vi "Load Messages and Populate Controls.vi"(8 "error in (no error)":errorcluster, 10 "Hierarchy":refnum<vi>, 11 "ListBox in":refnum<vi>) -> (0 "error out":errorcluster, 3 "Message map":map{string, T1}(c390))   [LabVIEW 2020, in "Sequencer.lvlib"]
uses:
  Sequencer.lvlib
  Controls/Ctl_MessageListElement.ctl
  PPL/HDH.ClassLoader.lvlibp
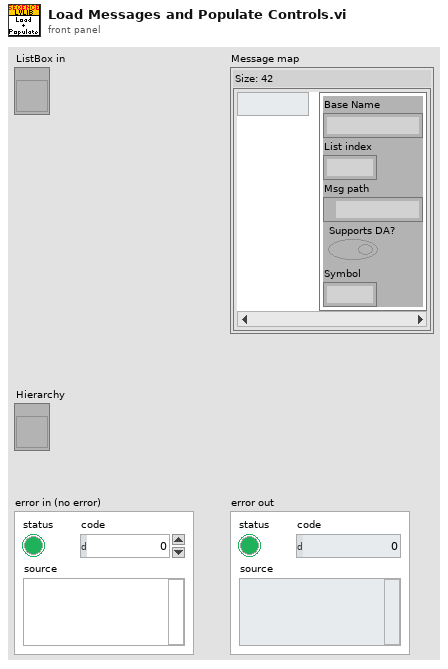
[diagram p1: front panel]
types:
  T1 = typedef "Sequencer.lvlib/Ctl_MessageListElement.ctl" = cluster{"Base Name":string, "List index":i32, "Msg path":path, "Supports DA?":bool, "Symbol":i32}
  T2 = typedef "HDH.ClassLoader.lvlibp/Ctl_Member Map.ctl" = map{string, T3}
  T3 = typedef "HDH.ClassLoader.lvlibp/HDH.ClassLoader_Member VI Info.ctl" = cluster{"qualified name":string, "path":path, "access scope":enum32{"invalid scope", "public", "private", "protected", "community"}, "is dynamic dispatch":bool}
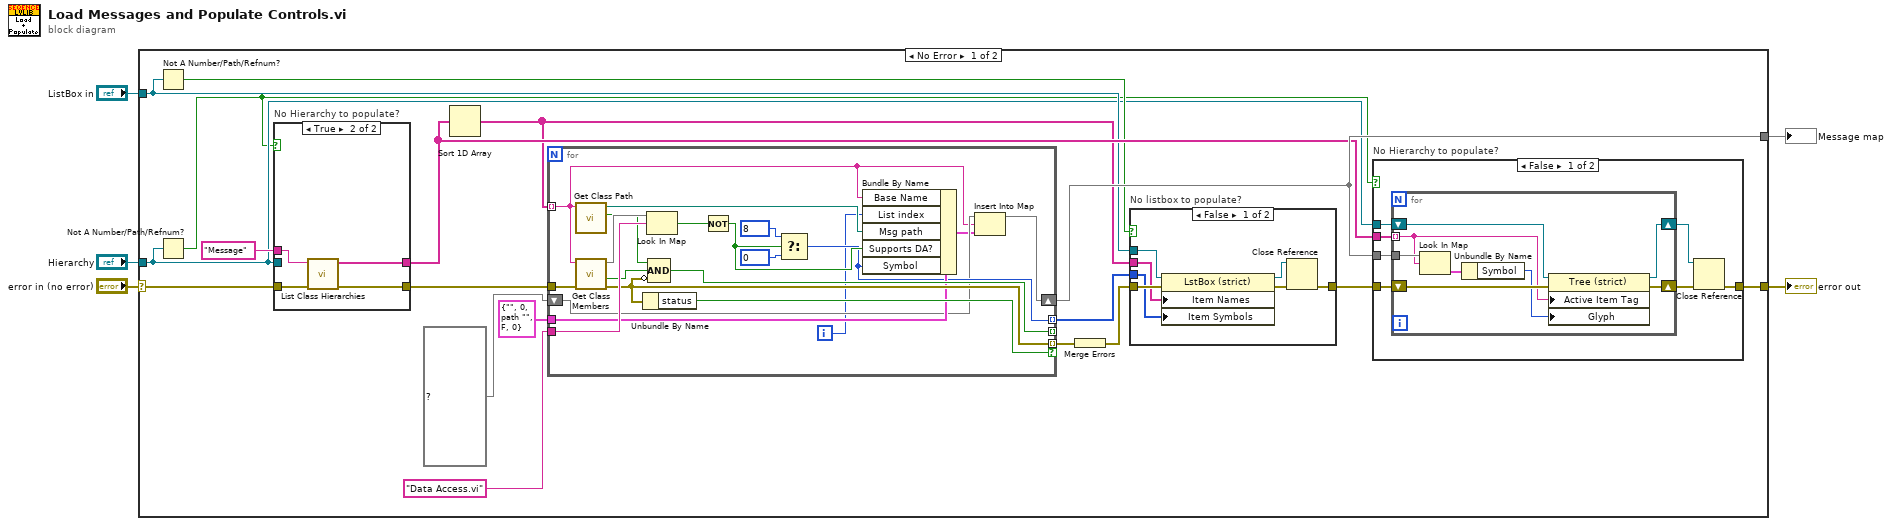
[diagram p0: block diagram]
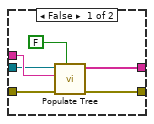
[diagram p3: hidden frame]
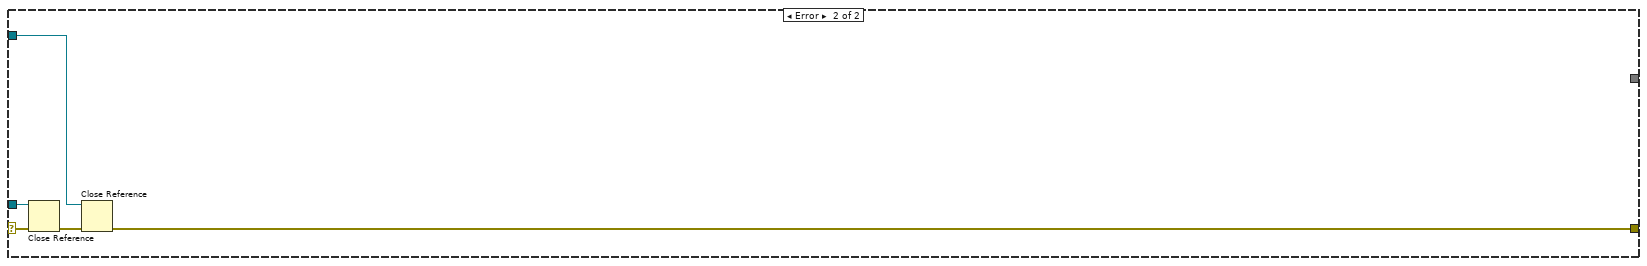
[diagram p5: hidden frame]
diagram:
  n1 = case shown="No Error" "error in (no error)" {
    selector: "error in (no error)" -> [w11 w82]
    tunnel: "Hierarchy" -> [w7 w79]
    tunnel: [w22 w81] -> w4
    tunnel: [w21 _] -> w3
    tunnel: "ListBox in" -> [w9 w78]
    frame No Error {
      n2 = Not A Number/Path/Refnum?(number/path/refnum=w9) -> (NaN/Path/Refnum?=w8:bool)
      n3 = Not A Number/Path/Refnum?(number/path/refnum=w7) -> (NaN/Path/Refnum?=w6:bool)
      n4 = case "No Hierarchy to populate?" shown="True" w6 {
        tunnel: [w44 w47] -> w20
        tunnel: [w43 w46] -> w13
        tunnel: w11 -> [w42 w49]
        tunnel: "Message" ("Hierarchy Filter(empty=all)") -> [w41 w48]
        tunnel: w7 -> [w40 _]
        frame False {
          n5 = call "Populate Tree.vi"("Close Reference?(T)"=FALSE, "error in (no error)"=w42, "Hierarchy Filter(empty=all)"=w41, "TreeControl in"=w40) -> ("error out"=w43:errorcluster, "Classes found"=w44:string[])  [unwired: 5 in, 1 out]
        }
        frame True {
          n6 = call "List Class Hierarchies.vi"("error in (no error)"=w49, "Hierarchy Filter(empty=all)"=w48) -> ("error out"=w46:errorcluster, "Classes found"=w47:string[])  [unwired: 6 in, 2 out]
        }
      }
      n7 = Sort 1D Array(array=w20) -> (sorted array=w15:string[])
      n8 = for {
        tunnel: w15 -> [w59] mode=indexing
        tunnel: w13 -> [w77]
        tunnel: "Data Access.vi" ("name or relative path") -> [w75]
        tunnel: [w70] -> w14 mode=indexing if=w73
        tunnel: [w69] -> _ mode=indexing
        tunnel: [w63] -> w16 mode=indexing
        tunnel: T1 {"Base Name"="", "List index"=0, "Msg path"=path "", "Supports DA?"=FALSE, "Symbol"=0} -> [w66]
        shift-right: [w61] -> w21
        shift-left: map{string, T1} {} ("map") -> [w62]
        i -> [w58]
        n9 = call "Get Class Path.vi"("Base Class Name"=w59) -> ("Success?"=w72:bool, "Path"=w65:path)  [unwired: 9 in]
        n10 = call "Get Class Members.vi"("error in (no error)"=w77, "Base Class Name"=w59) -> ("error out"=w70:errorcluster, "Success?"=w71:bool, "Member Map"=w76:T2)  [unwired: 7 in]
        n11 = Unbundle By Name(w70) -> ("status"=w73:bool)
        n12 = Look In Map(map=w76, key=w75) -> (key not found?=w74:bool)  [unwired: 1 in, 1 out]
        n13 = Compound Arithmetic op=AND(w72, w71, invert w70) -> (w69:bool)
        n14 = Not(x=w74) -> (.not. x?=w64:bool)
        n15 = Select(t=8, s=w64, f=0) -> (s? t:f=w63:i32)
        n16 = Bundle By Name(cluster=w66, "Base Name"=w59, "List index"=w58, "Msg path"=w65, "Supports DA?"=w64, "Symbol"=w63) -> (w60:T1)
        n17 = Insert Into Map(map in=w62, key=w59, value=w60) -> (map out=w61:map{string, T1})  [unwired: 2 out]
      }
      n18 = Merge Errors(w14) -> (w17:errorcluster)
      n19 = case "No listbox to populate?" shown="False" w8 {
        tunnel: [w56 w57] -> w23
        tunnel: w17 -> [w53 w57]
        tunnel: w16 -> [w52 _]
        tunnel: w15 -> [w51 _]
        tunnel: w9 -> [w50 _]
        frame False {
          n20 = property class="LstBox (strict)"(reference=w50, error in=w53, "Item Names"=w51, "Item Symbols"=w52) -> (reference out=w54:refnum<vi>, error out=w55:errorcluster)
          n21 = Close Reference(reference=w54, error in (no error)=w55) -> (error out=w56:errorcluster)
        }
        frame True {
        }
      }
      n22 = case "No Hierarchy to populate?" shown="False" w6 {
        tunnel: w23 -> [w29 w39]
        tunnel: [w27 w39] -> w22
        tunnel: w21 -> [w26 _]
        tunnel: w20 -> [w25 _]
        tunnel: w7 -> [w24 _]
        frame False {
          n23 = for {
            tunnel: w25 -> [w32] mode=indexing
            tunnel: w26 -> [w38]
            shift-right: [w35] -> w28
            shift-left: w24 -> [w36]
            shift-right: [w33] -> w30
            shift-left: w29 -> [w34]
            n24 = Look In Map(map=w38, key=w32) -> (value=w37:T1)  [unwired: 1 in, 1 out]
            n25 = Unbundle By Name(w37) -> ("Symbol"=w31:i32)
            n26 = property class="Tree (strict)"(reference=w36, error in=w34, "Active Item Tag"=w32, "Glyph"=w31) -> (reference out=w35:refnum<vi>, error out=w33:errorcluster)
          }
          n27 = Close Reference(reference=w28, error in (no error)=w30) -> (error out=w27:errorcluster)
        }
        frame True {
        }
      }
    }
    frame Error {
      n28 = Close Reference(reference=w79, error in (no error)=w82) -> (error out=w80:errorcluster)
      n29 = Close Reference(reference=w78, error in (no error)=w80) -> (error out=w81:errorcluster)
    }
  }
  "error out" <- w4
  "Message map" <- w3
